vi "Calibration pFC Data-old.vi"() -> ()   [LabVIEW 2014]
uses:
  <vilib>/Utility/file.llb/Read From Spreadsheet File (DBL).vi
  <vilib>/gmath/NumericalOptimization/Nonlinear Curve Fit LM formula string.vi
  <vilib>/Utility/file.llb/Write To Spreadsheet File (DBL).vi
  <vilib>/Analysis/NI_AALBase.lvlib
  <vilib>/gmath/NI_Gmath.lvlib
  <vilib>/Analysis/NI_AALPro.lvlib
panel:
  out "Selected xDNA (m51 count)":dbl[](array[numeric])
  out "Selected filt xDNA (m51 count)":dbl[](array[numeric])
  out "Selected xDNA (nm)":dbl[](array[numeric])
  in  "Final cut (s)":dbl=120.0
  out "Force (pN)":dbl
  out "read file path":path
  in  "Boolean":bool=TRUE
  out "Fraction (f-u)":dbl[](array[numeric])
  out "Funfold (%)":dbl
  out "Ffold (%)":dbl
  out "path":path
  in  "Fit?":bool
  in  "initial parameters":dbl[](array[numeric])=[200.0, 1100.0, 6.0, 500.0, 1120.0, 6.0]
  out "Laser Power (mV)":dbl
  out "Data rate (Hz)":dbl
  in  "Tab Control 2":enum32{"Folder", "File"}(tab)
  in  "Folder Path":path
  in  "file path (dialog if empty)":path
  in  "intervals for selected xDNA":i32=100
  out "Histogram: h(x)":i32[](array[numeric])
  out "Selected filt xDNA (nm)":dbl[](array[numeric])
  out "Selected Time (s)":dbl[](array[numeric]) format="%_7g"
  in  "Selected tf (s)":dbl=10.0
  in  "Selected ti (s)":dbl
  out "Time for total (s)":dbl[](array[numeric])
  out "Total Filtered xDNA (nm)":dbl[](array[numeric])
  out "Data rate for total (Hz)":dbl
  in  "Filter for total":T1(ring)=enum."Moving-window avg"
  in  "#Avg for total":i32=5
  in  "# of adjencent points":i32=5
  in  "Save?":bool
  out "Target QPD (V)":dbl
  out "Total xDNA (nm)":dbl[](array[numeric])
  in  "Filter for initial":T1(ring)
  out "Total Peak location (index)":i32[](array[numeric])
  out "Each first and end diff":dbl[](array[numeric])
  out "Total xDNA":dbl[][](array[numeric])
  out "cut-xDNA (nm)":dbl[](array[numeric])
  out "xDNA diff (i-(i+1))":dbl[](array[numeric])
  out "New stage moved index":i32[](array[numeric])
  in  "initial cut (s)":dbl=0.1
  out "Stage moved time index":i32[](array[numeric])
  out "Stage moved time (s)":dbl[](array[numeric])
  out "Time Array (s)":dbl[](array[numeric])
  out "xDNA (nm)":dbl[](array[numeric])
  in  "Tab Control":T2(tab)
  out "XY Graph 4":cluster{dbl[], "Filtered QPD data":dbl[]}[](graph)
  out "XY Graph":cluster{dbl[], dbl[]}(graph)
  out "Each first and end":dbl[](array[numeric])
  out "Each Section First and End index":i32[](array[numeric])
  out "XY Graph 2":cluster{dbl[], dbl[]}(graph)
  out "Waveform Graph":dbl[][](graph)
  out "XY Graph 3":cluster{dbl[], "Filtered QPD data":dbl[]}[](graph)
  out "XY Graph 5":cluster{dbl[], dbl[]}[](graph)
  out "Histogram Graph":T3(graph)
  out "best fit parameters":dbl[](array[numeric])
  out "dx transition (nm)":dbl
  out "XY Graph 7":cluster{dbl[], dbl[]}[](graph)
  in  "3nt binding signal (nm)":dbl=0.5
  out "XY Graph 6":T4(graph)
  out "Spatial Sampling Rate (1/nm)":dbl
  in  "intervals":i32=10
  out "Histogram Graph 2":T5(graph)
  in  "Pairwise?":bool
  out "Upper-Bound QPD radius (nm)":dbl=430.0
  in  "#Avg for initial":i32=25
  out "Data rate for initial (Hz)":dbl
  out "conversion factor (V/um)":dbl=0.75
  in  "Start point of Xbd for pFC (nm)":dbl=300.0
  in  "trap height(nm)":dbl=300.0
  # "try 350 for h=300\n      450 for h=0"
  # "20R xDNA~1100-1120 nm at 13.5 pN\nunfold dx=18 nm"
  # "0.09 for ~290mV"
  # "0.13 for 2800 mV"
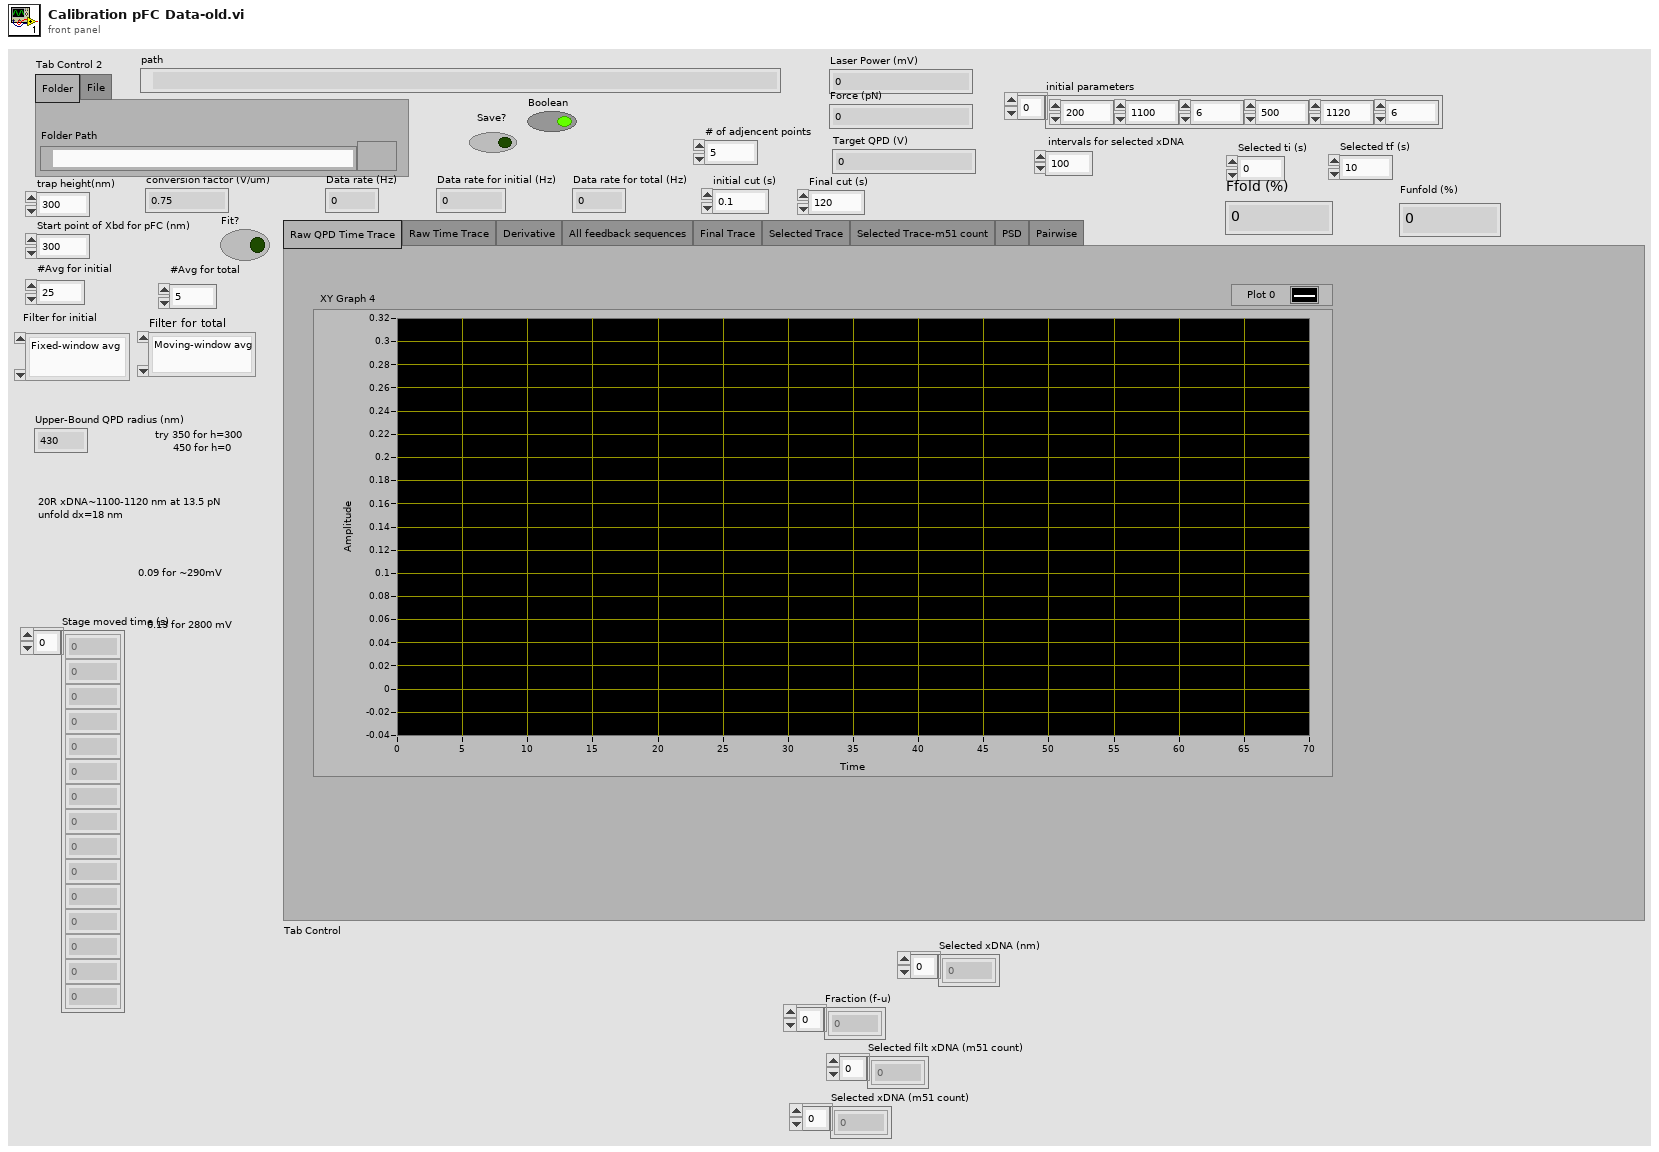
[diagram p1: front panel]
types:
  T1 = enum16{"Fixed-window avg", "Moving-window avg", "F+S-window avg", "S-G filter", "Fixed-window Median", "Moving-window Median "}
  T2 = enum32{"Raw QPD Time Trace", "Raw Time Trace", "Derivative", "All feedback sequences", "Final Trace", "Selected Trace", "Selected Trace-m51 count", "PSD", "Pairwise"}
  T3 = cluster{"X Values":dbl[], "best nonlinear fit":dbl[]}[]
  T4 = cluster{"Frequency (Hz)\n0,df, 2df,...(n/2-1)Fs":dbl[], "Power Spectrum (V^2 rms) (V^2/Hz)":dbl[]}
  T5 = cluster{"X Values":dbl[], "Histogram: h(x)":i32[]}
  T6 = cluster{"model":string, "Parameters":string[], "x":string}
  T7 = cluster{"initial amplitude":dbl, "initial center":dbl, "initial standard deviation":dbl, "offset":dbl}
  T8 = cluster{"X Values":dbl[], "best nonlinear fit":dbl[]}
  T9 = cluster{dbl[], "Power Spectrum (V^2 rms) (V^2/Hz)":dbl[]}
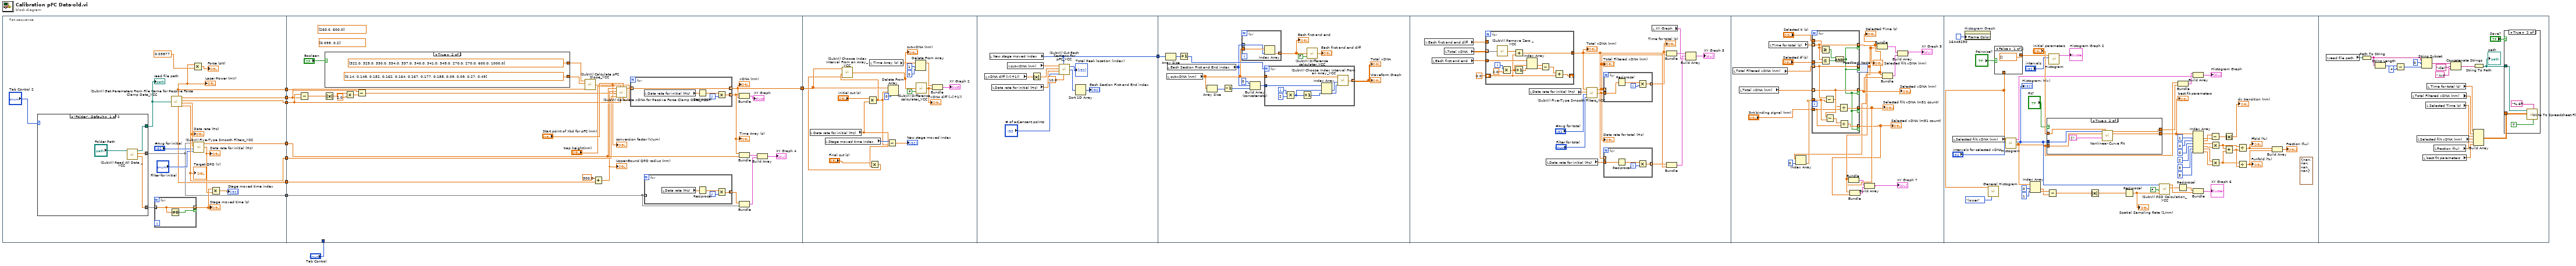
[diagram p0: block diagram]
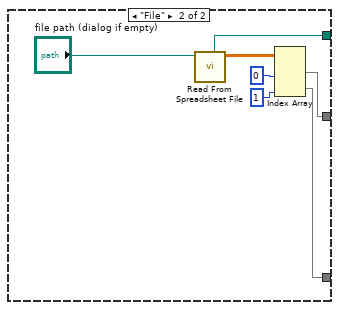
[diagram p2: hidden frame]
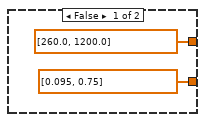
[diagram p3: hidden frame]
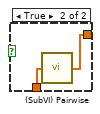
[diagram p4: hidden frame]
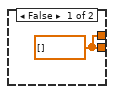
[diagram p5: hidden frame]
diagram:
  n1 = flat-sequence {
    tunnel: [w23] -> w10
    tunnel: [w28] -> w9
    tunnel: [w27] -> w8
    tunnel: [w26] -> w7
    tunnel: [w16] -> w3
    tunnel: [w13] -> w2
    tunnel: [w14] -> w1
    tunnel: "Tab Control" -> [_]
    tunnel: w7 -> [w64]
    tunnel: w8 -> [w65]
    tunnel: w9 -> [w59]
    tunnel: w10 -> [w57]
    tunnel: [w42] -> w5
    tunnel: w3 -> [w52]
    tunnel: w2 -> [w50]
    tunnel: w1 -> [w44]
    tunnel: w5 -> [w88]
    tunnel: [w106] -> w4
    tunnel: w4 -> [w120]
    frame #0 {
      n2 = case shown="\"Folder\", Default" "Tab Control 2" {
        tunnel: [w32 w34] -> w18
        tunnel: [w31 w33] -> w17
        tunnel: [w29 w35] -> w16
        frame "Folder", Default {
          n3 = call "(SubVI) Read All Data _YCC.vi"("Folder Path"="Folder Path") -> ("all moved time points"=w32:dbl[], "all QPD data"=w29:dbl[], "Last File Path"=w31:path)  [unwired: 4 in]
        }
        frame "File" {
          n4 = call-poly <vilib>:"Read From Spreadsheet File.vi"("file path (dialog if empty)"="file path (dialog if empty)") -> ("all rows"=w38:dbl[][], "new file path (Not A Path if cancelled)"=w33:path)  [unwired: 6 in, 3 out]
          n5 = Index Array(array=w38, index (col) #1=0 ("disabled index (col)"), index (col) #2=1 ("disabled index (col)")) -> (element #1=w35:dbl[], element #2=w34:dbl[])  [unwired: 2 in]
        }
      }
      "read file path" <- w17
      n6 = for {
        tunnel: [w40] -> w22 mode=indexing if=w41
        tunnel: w18 -> [w40] mode=indexing
        n7 = Not Equal To 0?(x=w40) -> (x != 0?=w41:bool)
      }
      "Stage moved time (s)" <- w22
      n8 = call "(SubVI) Get Paremeters From File Name for Passive Force Clamp Data_YCC.vi"("path"=w17) -> ("Target QPD (V)"=w27:dbl, "Jump (nm)"=w14:dbl, "Data rate (Hz)"=w25:dbl, "Moved position (um)"=w26:dbl, "Laser Power (mV)"=w13:dbl, "Center position (um)"=w28:dbl)  [unwired: 2 in]
      "Target QPD (V)" <- w27
      "Data rate (Hz)" <- w25
      "Laser Power (mV)" <- w13
      n9 = Multiply(x=w13, y=0.03877) -> (x*y=→"Force (pN)":dbl)
      n10 = call "(SubVI) Five-Type Smooth Filters_YCC.vi"("Filter type"="Filter for initial", "Avg points"="#Avg for initial", "Sampling rate (Hz)"=w25, "QPD data"=w16) -> ("Sampling rate after filtering (Hz)"=w21:dbl, "Filtered QPD data"=w23:dbl[])  [unwired: 1 in]
      "Data rate for initial (Hz)" <- w21
      n11 = Multiply(x=w22, y=w21) -> (x*y=→"Stage moved time index":dbl[])
    }
    frame #1 {
      (unwired) dbl[] [0.095, 0.2] ("Slope")
      (unwired) dbl[] [260.0, 600.0] ("power")
      n12 = Subtract(x=w64, y=w59) -> (x-y=w63:dbl)
      n13 = Absolute Value(x=w63) -> (abs(x)=w61:dbl)
      n14 = case shown="True" "Boolean" {
        tunnel: [dbl[] [260.0, 1200.0] ("power") dbl[] [322.0, 325.0, 330.0, 334.0, 337.0, 340.0, 341.0, 349.0, 270.0, 270.0, 600.0, 1000.0] ("power")] -> w48
        tunnel: [dbl[] [0.095, 0.75] ("Slope") dbl[] [0.14, 0.148, 0.152, 0.162, 0.164, 0.167, 0.177, 0.188, 0.09, 0.09, 0.27, 0.49] ("Slope")] -> w47
        frame False {
        }
        frame True {
        }
      }
      n15 = Multiply(x=w61, y=2.0) -> (x*y=w60:dbl)
      n16 = Subtract(x=w59, y=w60) -> (x-y=w58:dbl)
      n17 = call "(SubVI) Calculate pFC Slope_YCC.vi"("given-power"=w50, "Slope"=w47, "power"=w48) -> ("Cal-slope (V/um)"=w49:dbl)  [unwired: 3 in]
      "conversion factor (V/um)" <- w49
      n18 = Add(x=300.0, y=w44) -> (x+y=w43:dbl)
      "Upper-Bound QPD radius (nm)" <- w43
      n19 = call "(SubVI) Calculate xDNA for Passive Force Clamp Data_YCC.vi"("conversion factor (V/um)"=w49, "Start point of Xbd for pFC (nm)"="Start point of Xbd for pFC (nm)", "Move to (um)"=w64, "trap height(nm)"="trap height(nm)", "QPD center value (V)"=w65, "Stage center point (um)"=w58, "Target QPD radius (nm)"=w43, "QPD Array (V)"=w57) -> ("xDNA (nm)"=w69:dbl[])  [unwired: 1 in, 2 out]
      n20 = for {
        tunnel: w69 -> [w78] mode=indexing
        tunnel: [w79] -> w56 mode=indexing
        tunnel: [w78] -> w42 mode=indexing
        i -> [w82]
        n21 = local read "Data rate for initial (Hz)"() -> (w81:dbl)
        n22 = Reciprocal(x=w81) -> (1/x=w80:dbl)
        n23 = Multiply(x=w80, y=w82) -> (x*y=w79:dbl)
      }
      "xDNA (nm)" <- w42
      "Time Array (s)" <- w56
      n24 = for {
        tunnel: w52 -> [_] mode=indexing
        tunnel: [w74] -> w51 mode=indexing
        i -> [w75]
        n25 = local read "Data rate (Hz)"() -> (w77:dbl)
        n26 = Reciprocal(x=w77) -> (1/x=w76:dbl)
        n27 = Multiply(x=w76, y=w75) -> (x*y=w74:dbl)
      }
      n28 = Bundle(w56, w42) -> (→"XY Graph":cluster{dbl[], dbl[]})  [unwired: 1 in]
      n29 = Bundle(w56, "Filtered QPD data"=w57) -> (w53:cluster{dbl[], "Filtered QPD data":dbl[]})  [unwired: 1 in]
      n30 = Bundle(w51, "all rows"=w52) -> (w54:cluster{dbl[], "all rows":dbl[]})  [unwired: 1 in]
      n31 = Build Array(w53, w54) -> (→"XY Graph 4":cluster{dbl[], "all rows":dbl[]}[])
    }
    frame #2 {
      n32 = local read "Data rate for initial (Hz)"() -> (w87:dbl)
      n33 = local read "Stage moved time index"() -> (w90:i32[])
      n34 = Multiply(x="initial cut (s)", y=w87) -> (x*y=w85:dbl)
      n35 = local read "Time Array (s)"() -> (w99:dbl[])
      n36 = Multiply(x="Final cut (s)", y=w87) -> (x*y=w84:dbl)
      n37 = call "(SubVI) Choose Index Interval From an Array_YCC.vi"("End index"=w84, "Start index"=w85, "array"=w88) -> ("Array out"=w83:dbl[])  [unwired: 3 in]
      "cut-xDNA (nm)" <- w83
      n38 = Subtract(x=w90, y=w85) -> (x-y=→"New stage moved index":dbl[])
      n39 = Delete From Array(array=w88, length=w85, index=0) -> ()  [unwired: 2 out]
      n40 = Delete From Array(array=w99, length=1, index=0) -> (array with subset deleted=w95:dbl[])  [unwired: 1 out]
      n41 = call "(SubVI) Difference calculater_YCC.vi"("T= (i+1)-i\nF=i-(i+1)"=FALSE ("T= (i+1)-i\nF=i-(i+1)"), "Array in"=w83) -> ("Diff"=w94:dbl[])  [unwired: 3 in]
      "xDNA diff (i-(i+1))" <- w94
      n42 = Bundle("Time Array (s)"=w95, "Diff"=w94) -> (→"XY Graph 2":cluster{"Time Array (s)":dbl[], "Diff":dbl[]})  [unwired: 1 in]
    }
    frame #3 {
      n43 = local read "xDNA diff (i-(i+1))"() -> (w103:dbl[])
      n44 = local read "New stage moved index"() -> (w106:i32[])
      n45 = local read "Data rate for initial (Hz)"() -> (w107:dbl)
      n46 = local read "cut-xDNA (nm)"() -> (w108:dbl[])
      n47 = Absolute Value(x=w103) -> (abs(x)=w102:dbl[])
      n48 = call "(SubVI) Cut Each Sections For pFC_YCC.vi"("xDNA"=w108, "Initial guess locations"=w106, "Diff (i-i+1)"=w102, "Data Rate (Hz)"=w107, "threshold y"=10.0, "# of adjencent points"="# of adjencent points") -> ("Total Peak location (index)"=→"Total Peak location (index)":i32[], "Each Section First and End index"=w101:i32[])  [unwired: 1 in]
      n49 = Sort 1D Array(array=w101) -> (sorted array=→"Each Section First and End index":i32[])
    }
    frame #4 {
      n50 = Array Size(array=w120) -> (size(s)=w119:i32)
      n51 = local read "cut-xDNA (nm)"() -> (w111:dbl[])
      n52 = local read "Each Section First and End index"() -> (w112:i32[])
      n53 = Increment(x=w119) -> (x+1=w118:i32)
      n54 = Array Size(array=w111) -> (size(s)=w115:i32)
      n55 = Decrement(x=w115) -> (x-1=w114:i32)
      n56 = for {
        tunnel: w112 -> [w124] mode=indexing
        tunnel: w111 -> [w125]
        tunnel: [w123] -> w110 mode=indexing
        n57 = Index Array(array=w125, index=w124) -> (element=w123:dbl)
      }
      "Each first and end" <- w110
      n58 = Build Array (concatenate)(0, w112, w114) -> (w116:i32[])
      n59 = for {
        N: w118 -> [_]
        tunnel: w111 -> [w134]
        tunnel: w116 -> [w133]
        tunnel: [w127] -> w113 mode=indexing
        i -> [w126]
        n60 = Multiply(x=w126, y=2) -> (x*y=w129:i32)
        n61 = Increment(x=w129) -> (x+1=w128:i32)
        n62 = Index Array(array=w133, index #1=w129, index #2=w128) -> (element #1=w132:i32, element #2=w131:i32)
        n63 = call "(SubVI) Choose Index Interval From an Array_YCC.vi"("End index"=w131, "Start index"=w132, "array"=w134) -> ("Array out"=w127:dbl[])  [unwired: 3 in]
      }
      "Waveform Graph" <- w113
      "Total xDNA" <- w113
      n64 = call "(SubVI) Difference calculater_YCC.vi"("T= (i+1)-i\nF=i-(i+1)"=FALSE ("T= (i+1)-i\nF=i-(i+1)"), "Array in"=w110) -> ("Diff"=→"Each first and end diff":dbl[])  [unwired: 3 in]
    }
    frame #5 {
      n65 = local read "Each first and end diff"() -> (w151:dbl[])
      n66 = local read "Each first and end"() -> (w150:dbl[])
      n67 = local read "Total xDNA"() -> (w146:dbl[][])
      n68 = for {
        tunnel: w146 -> [w171] mode=indexing
        tunnel: w151 -> [_]
        tunnel: [w172] -> w145 mode=concatenating
        tunnel: w150 -> [w165]
        shift-right: [w161] -> _
        shift-left: 0.0 -> [w160]
        i -> [w168]
        n69 = call "(SubVI) Remove Zero _YCC.vi"("Array in"=w171) -> ("Array out"=w170:dbl[])  [unwired: 4 in]
        n70 = Multiply(x=w168, y=2.0) -> (x*y=w167:dbl)
        n71 = Add(x=w170, y=w160) -> (x+y=w172:dbl[])
        n72 = Increment(x=w167) -> (x+1=w166:dbl)
        n73 = Index Array(array=w165, index #1=w167, index #2=w166) -> (element #1=w164:dbl, element #2=w163:dbl)
        n74 = Subtract(x=w164, y=w163) -> (x-y=w162:dbl)
        n75 = Add(x=w162, y=w160) -> (x+y=w161:dbl)
      }
      "Total xDNA (nm)" <- w145
      n76 = local read "Data rate for initial (Hz)"() -> (w144:dbl)
      n77 = local read "Data rate for initial (Hz)"() -> (w148:dbl)
      n78 = call "(SubVI) Five-Type Smooth Filters_YCC.vi"("Filter type"="Filter for total", "Avg points"="#Avg for total", "Sampling rate (Hz)"=w144, "QPD data"=w145) -> ("Sampling rate after filtering (Hz)"=w138:dbl, "Filtered QPD data"=w139:dbl[])  [unwired: 1 in]
      "Data rate for total (Hz)" <- w138
      "Total Filtered xDNA (nm)" <- w139
      n79 = for {
        tunnel: w138 -> [w155]
        tunnel: [w153] -> w137 mode=indexing
        tunnel: w139 -> [_] mode=indexing
        i -> [w152]
        n80 = Reciprocal(x=w155) -> (1/x=w154:dbl)
        n81 = Multiply(x=w154, y=w152) -> (x*y=w153:dbl)
      }
      "Time for total (s)" <- w137
      n82 = for {
        tunnel: w145 -> [_] mode=indexing
        tunnel: w148 -> [w159]
        tunnel: [w157] -> w147 mode=indexing
        i -> [w156]
        n83 = Reciprocal(x=w159) -> (1/x=w158:dbl)
        n84 = Multiply(x=w158, y=w156) -> (x*y=w157:dbl)
      }
      n85 = local read "XY Graph"() -> (w135:cluster{dbl[], dbl[]})
      n86 = Bundle(w137, "Filtered QPD data"=w139) -> (w140:cluster{dbl[], "Filtered QPD data":dbl[]})  [unwired: 1 in]
      n87 = Bundle(w147, w145) -> (w141:cluster{dbl[], dbl[]})  [unwired: 1 in]
      n88 = Build Array(w140, w141, w135) -> (→"XY Graph 3":cluster{dbl[], "Filtered QPD data":dbl[]}[])
    }
    frame #6 {
      n89 = local read "Total Filtered xDNA (nm)"() -> (w184:dbl[])
      n90 = local read "Total xDNA (nm)"() -> (w189:dbl[])
      n91 = local read "Time for total (s)"() -> (w192:dbl[])
      n92 = feedback #1() -> (w173:dbl[])  [unwired: 1 in]
      "Selected filt xDNA (nm)" <- w173
      n93 = Index Array(array=w173, index=0) -> (element=w182:dbl)
      n94 = for {
        tunnel: w192 -> [w205] mode=indexing
        tunnel: [w201] -> w174 mode=indexing if=w193
        tunnel: w184 -> [w201] mode=indexing
        tunnel: [w205] -> w180 mode=indexing if=w193
        tunnel: "Selected ti (s)" -> [w206]
        tunnel: "Selected tf (s)" -> [w204]
        tunnel: w189 -> [w200] mode=indexing
        tunnel: [w200] -> w188 mode=indexing if=w193
        tunnel: w182 -> [w199]
        tunnel: "3nt binding signal (nm)" -> [w196]
        tunnel: [w195] -> w179 mode=indexing if=w193
        tunnel: [w194] -> w177 mode=indexing if=w193
        n95 = Greater Or Equal?(x=w205, y=w206) -> (x >= y?=w203:bool)
        n96 = Less Or Equal?(x=w205, y=w204) -> (x <= y?=w202:bool)
        n97 = Subtract(x=w201, y=w199) -> (x-y=w198:dbl)
        n98 = Subtract(x=w200, y=w199) -> (x-y=w197:dbl)
        n99 = And(x=w203, y=w202) -> (x .and. y?=w193:bool)
        n100 = Divide(x=w198, y=w196) -> (x/y=w195:dbl)
        n101 = Divide(x=w197, y=w196) -> (x/y=w194:dbl)
      }
      "Selected Time (s)" <- w180
      "Selected xDNA (nm)" <- w188
      "Selected filt xDNA (m51 count)" <- w179
      "Selected xDNA (m51 count)" <- w177
      n102 = Bundle(w180, w179) -> (w178:cluster{dbl[], dbl[]})  [unwired: 1 in]
      n103 = Bundle(w180, w177) -> (w176:cluster{dbl[], dbl[]})  [unwired: 1 in]
      n104 = feedback-in #1(w174) -> ()
      n105 = Build Array(w178, w176) -> (→"XY Graph 7":cluster{dbl[], dbl[]}[])
      n106 = Bundle(w180, w173) -> (w186:cluster{dbl[], dbl[]})  [unwired: 1 in]
      n107 = Bundle(w180, w188) -> (w185:cluster{dbl[], dbl[]})  [unwired: 1 in]
      n108 = Build Array(w186, w185) -> (→"XY Graph 5":cluster{dbl[], dbl[]}[])
    }
    frame #7 {
      (unwired) T7 {"initial amplitude"=nan, "initial center"=nan, "initial standard deviation"=nan, "offset"=nan} ("initial guess")
      n109 = local read "Selected filt xDNA (nm)"() -> (w208:dbl[])
      n110 = property on="Histogram Graph" class="XYGraph (strict)"("Frame Color"=u32 16448250) -> ()  [unwired: 2 in, 2 out]
      n111 = call <vilib>:"General Histogram.vi"("X"=w208, "inclusion"=enum32{"lower", "upper"}."lower") -> ()  [unwired: 9 in, 5 out]
      n112 = case shown="False" "Pairwise?" {
        tunnel: w208 -> [_ w258]
        tunnel: [dbl[] [] ("Pairwise") w257] -> w212
        frame False {
        }
        frame True {
          n113 = call "(SubVI) Pairwise.vi"("Data"=w258) -> ("Pairwise"=w257:dbl[])  [unwired: 4 in]
        }
      }
      n114 = call <vilib>:"Histogram.vi"("intervals"="intervals for selected xDNA", "X"=w208) -> ("X Values"=w242:dbl[], "Histogram: h(x)"=w244:i32[], "Histogram Graph"=w239:T5)  [unwired: 6 in, 1 out]
      "Histogram: h(x)" <- w244
      n115 = Index Array(array=w242, index #1=0 ("index"), index #2=1 ("index")) -> (element #1=w250:dbl, element #2=w251:dbl)
      n116 = case shown="True" "Fit?" {
        tunnel: w244 -> [_ w264]
        tunnel: "initial parameters" -> [_ w263]
        tunnel: w242 -> [_ w262]
        tunnel: [w259 w261] -> w241
        tunnel: [w259 w260] -> w237
        frame False {
          w259 = dbl[] [] ("best nonlinear fit")
        }
        frame True {
          n117 = call-poly <vilib>:"Nonlinear Curve Fit.vi"("Y"=w264, "initial parameters"=w263, "X"=w262, "model description"=T6 {"model"="a1*exp(-((u-a2)/a3)^2)+a4*exp(-((u-a5)/a6)^2)", "Parameters"=["a1", "a2", "a3", "a4", "a5", "a6"], "x"="u"}) -> ("best nonlinear fit"=w261:dbl[], "best fit parameters"=w260:dbl[])  [unwired: 7 in, 3 out]
        }
      }
      "best fit parameters" <- w237
      n118 = Subtract(x=w251, y=w250) -> (x-y=w249:dbl)
      n119 = call <vilib>:"Histogram.vi"("intervals"="intervals", "X"=w212) -> ("Histogram Graph"=→"Histogram Graph 2":T5)  [unwired: 6 in, 3 out]
      n120 = Absolute Value(x=w249) -> (abs(x)=w248:dbl)
      n121 = Reciprocal(x=w248) -> (1/x=w247:dbl)
      "Spatial Sampling Rate (1/nm)" <- w247
      n122 = call "(SubVI) PSD Calculation_YCC.vi"("sampling frequency (Hz)"=w247, "T=NI made PSD\nF=YCC made PSD"=FALSE ("T=NI made PSD\nF=YCC made PSD"), "QPD data"=w244) -> ("Frequency (Hz)\n0,df, 2df,...(n/2-1)Fs"=w229:dbl[], "Power Spectrum (V^2 rms) (V^2/Hz)"=w246:dbl[])  [unwired: 3 in]
      n123 = Reciprocal(x=w229) -> (1/x=w228:dbl[])
      n124 = Bundle("X Values"=w242, "best nonlinear fit"=w241) -> (w238:T8)  [unwired: 1 in]
      n125 = Index Array(array=w237, index #1=1 ("index"), index #2=4 ("index"), index #3=0 ("index"), index #4=2 ("index"), index #5=3 ("index"), index #6=5 ("index")) -> (element #1=w233:dbl, element #2=w234:dbl, element #3=w223:dbl, element #4=w222:dbl, element #5=w221:dbl, element #6=w220:dbl)
      n126 = Build Array(w238, w239) -> (→"Histogram Graph":T3)
      n127 = Bundle(w228, "Power Spectrum (V^2 rms) (V^2/Hz)"=w246) -> (→"XY Graph 6":T9)  [unwired: 1 in]
      n128 = Subtract(x=w234, y=w233) -> (x-y=w232:dbl)
      n129 = Multiply(x=w223, y=w222) -> (x*y=w219:dbl)
      n130 = Multiply(x=w221, y=w220) -> (x*y=w217:dbl)
      n131 = Absolute Value(x=w232) -> (abs(x)=→"dx transition (nm)":dbl)
      n132 = Add(x=w219, y=w217) -> (x+y=w218:dbl)
      n133 = Divide(x=w219, y=w218) -> (x/y=w216:dbl)
      "Ffold (%)" <- w216
      n134 = Divide(x=w217, y=w218) -> (x/y=w215:dbl)
      "Funfold (%)" <- w215
      n135 = Build Array(w216, w215) -> (→"Fraction (f-u)":dbl[])
    }
    frame #8 {
      n136 = local read "read file path"() -> (w278:path)
      n137 = Path To String(path=w278) -> (string=w273:string)
      n138 = String Length(string=w273) -> (length=w277:i32)
      n139 = Subtract(x=w277, y=4) -> (x-y=w275:i32)
      n140 = local read "Total Filtered xDNA (nm)"() -> (w282:dbl[])
      n141 = local read "Selected filt xDNA (nm)"() -> (w280:dbl[])
      n142 = String Subset(string=w273, offset (0)=0, length (rest)=w275) -> (substring=w272:string)
      n143 = local read "best fit parameters"() -> (w266:dbl[])
      n144 = local read "Selected Time (s)"() -> (w279:dbl[])
      n145 = local read "Time for total (s)"() -> (w283:dbl[])
      n146 = local read "Fraction (f-u)"() -> (w267:dbl[])
      n147 = Concatenate Strings(w272, "-Cal" ("string"), ".txt" ("string")) -> (w269:string)
      n148 = String To Path(string=w269) -> (path=w268:path)
      "path" <- w268
      n149 = Build Array(w283, w282, w279, w280, w267, w266) -> (w281:dbl[][])
      n150 = case shown="True" "Save?" {
        tunnel: w281 -> [_ w286]
        tunnel: w268 -> [_ w285]
        frame False {
        }
        frame True {
          n151 = call-poly <vilib>:"Write To Spreadsheet File.vi"("transpose? (no:F)"=TRUE, "format (%.3f)"="%.6f", "2D data"=w286, "file path (dialog if empty)"=w285) -> ()  [unwired: 4 in, 1 out]
        }
      }
    }
  }
